vi "Read Dependency items.vi"(11 "CDependencyList in":refnum<class "CDependencyList.lvclass">) -> (2 "Dependency items":refnum<class "ILabVIEWItem.lvclass">[](array[class]), 3 "CDependencyList out":refnum<class "CDependencyList.lvclass">)   [LabVIEW 2020, in "DependencyInspection.lvlib" / "CDependencyList.lvclass"]
uses:
  CDependencyList.lvclass
  obj/Addons/LabVIEWObjectInterfaces.lvlibp/LabVIEWObjectInterfaces/ILabVIEWItem/ILabVIEWItem.lvclass
  CDependencyList.lvclass/CDependencyList.ctl
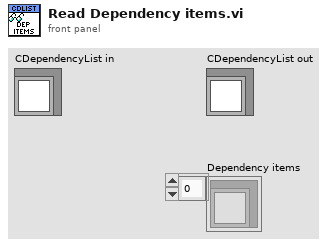
[diagram p1: front panel]
types:
  T1 = typedef "DependencyInspection.lvlib/CDependencyList.lvclass/DependencyListRef.ctl" = refnum<data-value>
  T2 = typedef "DependencyInspection.lvlib/CDependencyList.lvclass/DependencyList.ctl" = map{string, refnum<class "ILabVIEWItem.lvclass">}
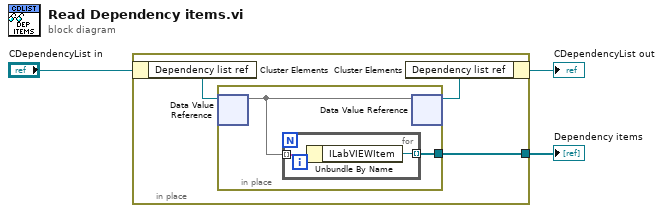
[diagram p0: block diagram]
diagram:
  n1 = in-place {
    in-place-border: [w4] -> w1
    n2 = in-place-cluster #1("CDependencyList in") -> ("Dependency list ref"=w6:T1)
    n3 = in-place {
      in-place-border: [w7] -> w4
      n4 = in-place-dvr #2(w6) -> (w8:T2)  [unwired: 1 out]
      n5 = for {
        tunnel: w8 -> [w10] mode=indexing
        tunnel: [w9] -> w7 mode=indexing
        n6 = Unbundle By Name(w10) -> ("ILabVIEWItem"=w9:refnum<class "ILabVIEWItem.lvclass">)
      }
      n7 = in-place-dvr #2(w8) -> (w5:T1)  [unwired: 1 out]
    }
    n8 = in-place-cluster #1("Dependency list ref"=w5) -> (→"CDependencyList out":refnum<class "CDependencyList.lvclass">)
  }
  "Dependency items" <- w1
